vi "StackerManualOverride.vi"(9 "Shut Off No.":i32, 10 "Stacker Manual":dbl, 11 "Stacker Output":dbl) -> (2 "Stacker Off?":bool, 3 "Final Stacker Output":dbl)   [LabVIEW 2014]
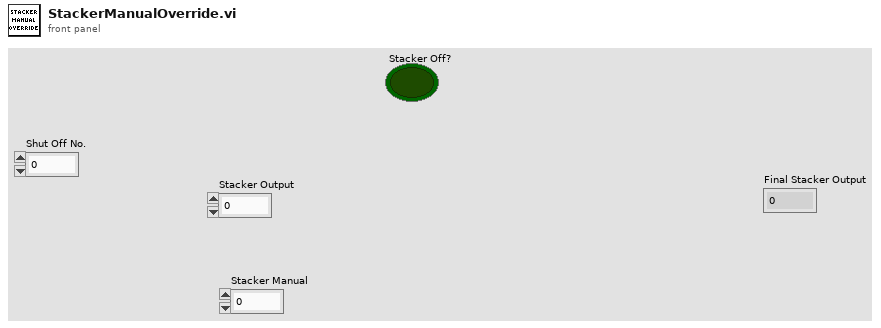
[diagram p1: front panel]
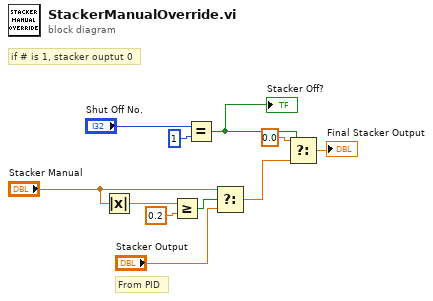
[diagram p0: block diagram]
diagram:
  # "if # is 1, stacker ouptut 0"
  # "From PID"
  n1 = Absolute Value(x="Stacker Manual") -> (abs(x)=w8:dbl)
  n2 = Greater Or Equal?(x=w8, y=0.2) -> (x >= y?=w10:bool)
  n3 = Equal?(x="Shut Off No.", y=1) -> (x = y?=w1:bool)
  "Stacker Off?" <- w1
  n4 = Select(t="Stacker Manual", s=w10, f="Stacker Output") -> (s? t:f=w4:dbl)
  n5 = Select(t=0.0, s=w1, f=w4) -> (s? t:f=→"Final Stacker Output":dbl)
